vi "Set Hidden.vi"(8 "error in (no error)":errorcluster, 11 "Panel in":refnum<class "Panel.lvclass">) -> (0 "error out":errorcluster, 3 "Panel out":refnum<class "Panel.lvclass">)   [LabVIEW 2020, in "OOPanel.lvlib" / "Panel.lvclass"]
uses:
  <vilib>/IlluminatedG/IG OOPanel/OOPanel/Panel/Panel.lvclass
  <vilib>/IlluminatedG/IG OOPanel/OOPanel/Panel/Visibility State.ctl
  <vilib>/IlluminatedG/IG OOPanel/OOPanel/OOPanel.lvlib
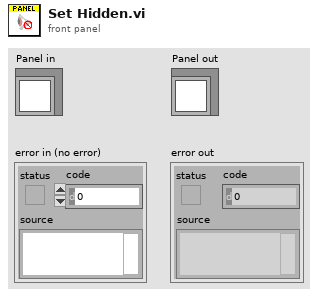
[diagram p1: front panel]
types:
  T1 = typedef "OOPanel.lvlib/Visibility State.ctl" = enum16{"Idle", "Closed", "Hidden", "Visible", "Subpanel"}
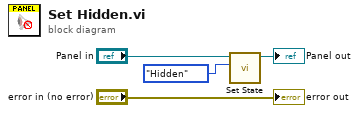
[diagram p0: block diagram]
diagram:
  n1 = call <vilib>:"Set State.vi"("State"=Visibility_State."Hidden", "Panel in"="Panel in") -> ("Panel out"=→"Panel out":refnum<class "Panel.lvclass">)  [unwired: 8 in, 1 out]
  "error out" <- "error in (no error)"
